vi "LED.vi"(9 "Control_State":T1, 10 "Length":dbl, 11 "Iteration_Num":dbl) -> (3 "Output_Array":u32[](array[numeric]))   [LabVIEW 2020]
uses:
  LED_Control_States.ctl
  <vilib>/numeric/Random Number (Range) U64.vi
  af1e4812-ce9e-4321-a641-5b8f74c4ca52.vi
  <vilib>/numeric/sub_Random U32.vi
panel:
  in  "Numbers":dbl[](array[numeric])=[2.0, 4.0, 100.0, 30.0, 2.0, 6.0]
  in  "colors":u32[](array[colorbox])=[16712704, 1507583, 65302]
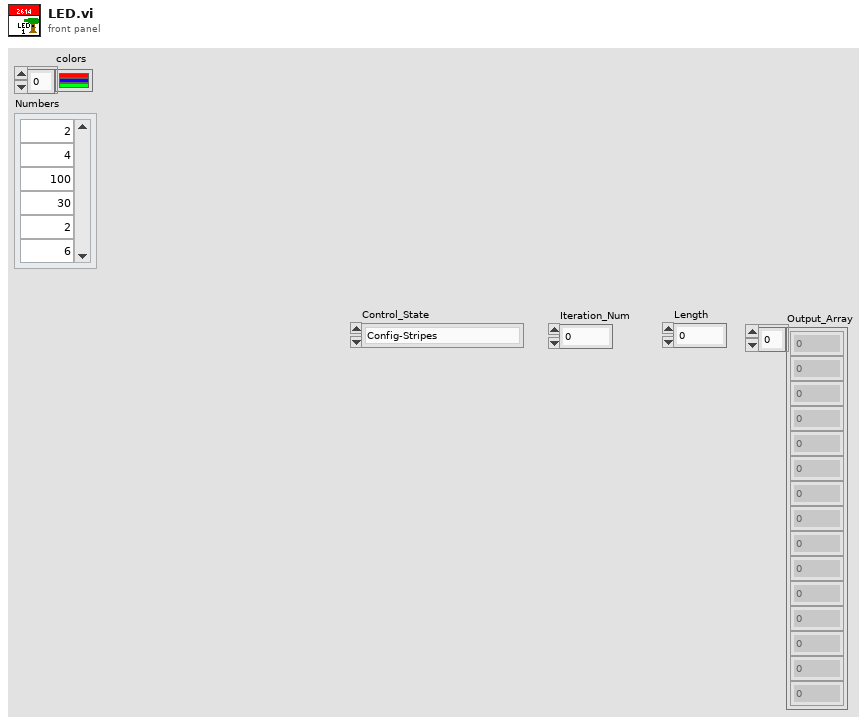
[diagram p1: front panel]
types:
  T1 = typedef "LED_Control_States.ctl" = enum16{"Config-Stripes", "swapperlines", "Rand", "Solid", "Flash-S", "Gradyent", "Move-Stripes", "Org-Rand", "Move-Point-Tail", "Flames", "Fade", "Alt-Colors"}
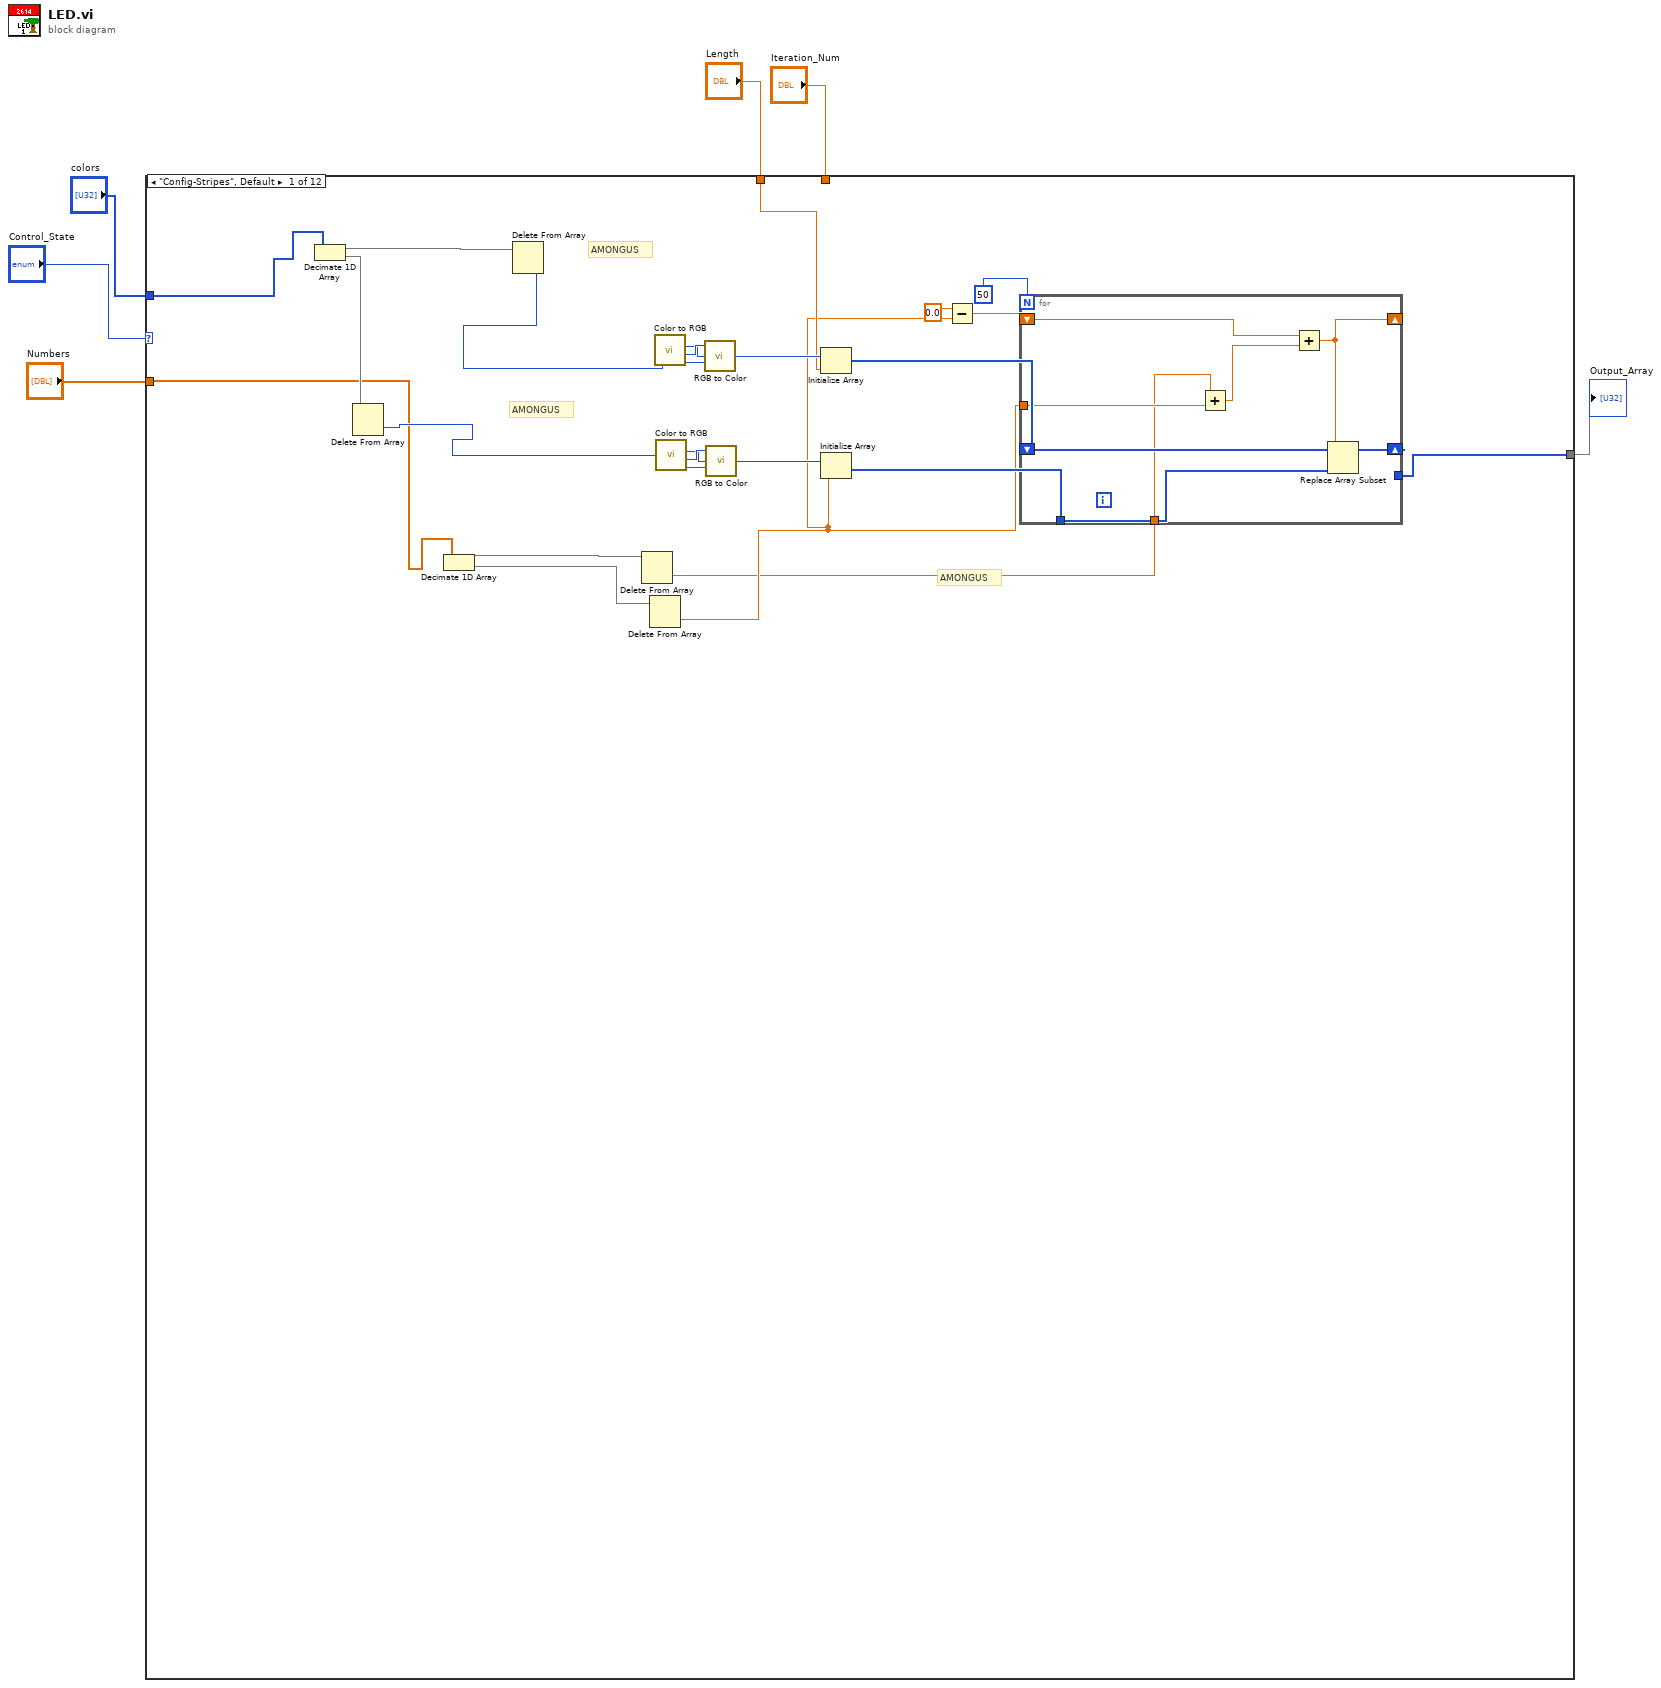
[diagram p0: block diagram]
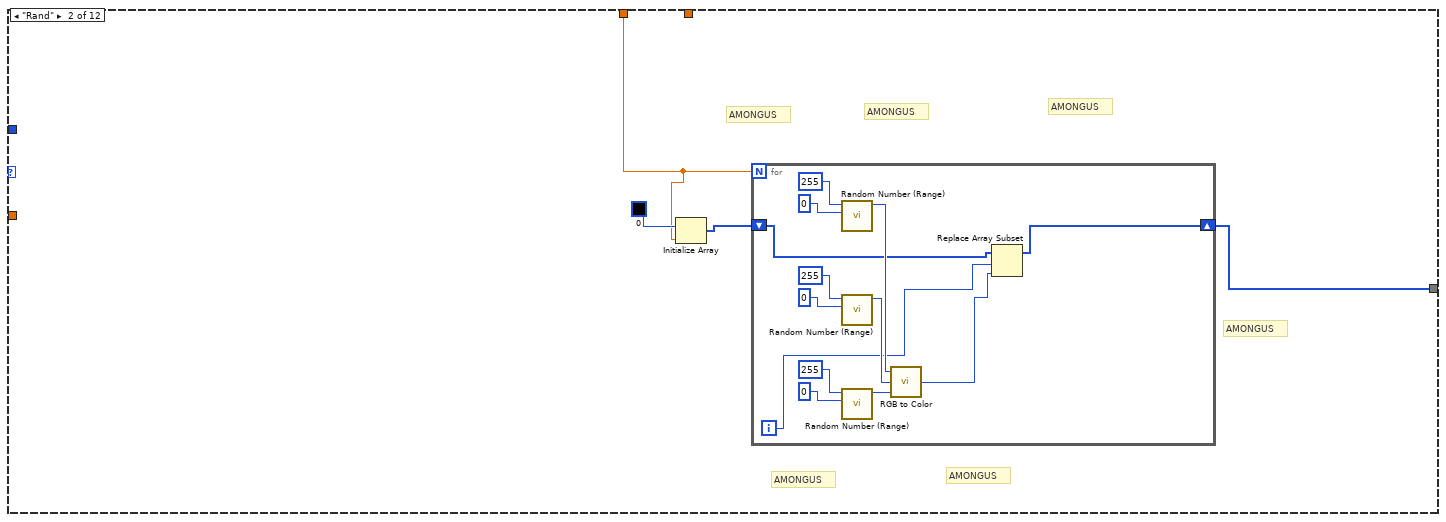
[diagram p2: hidden frame]
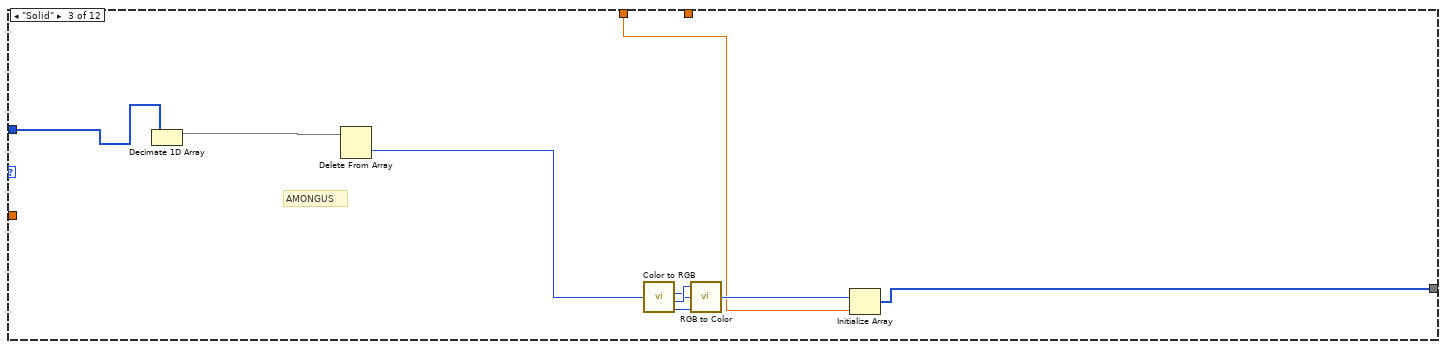
[diagram p3: hidden frame]
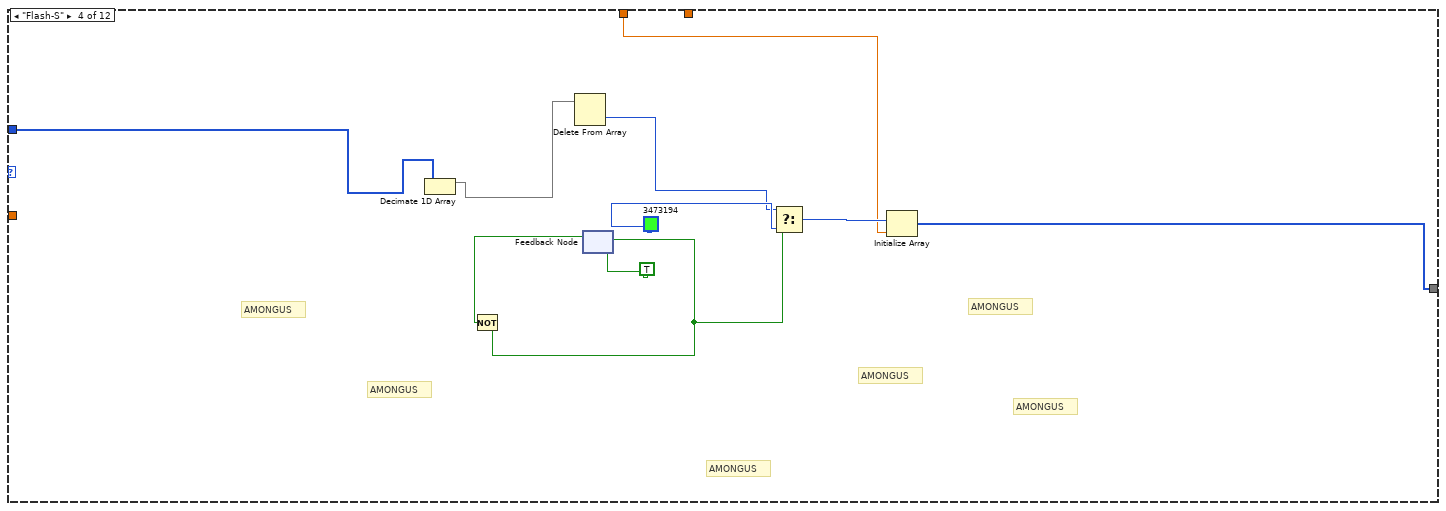
[diagram p4: hidden frame]
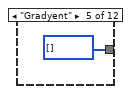
[diagram p5: hidden frame]
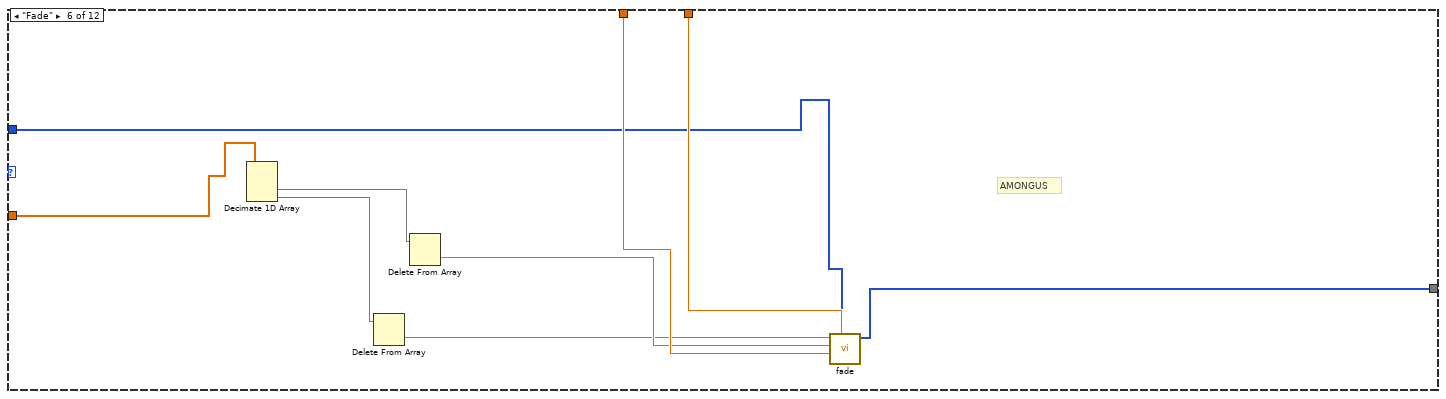
[diagram p6: hidden frame]
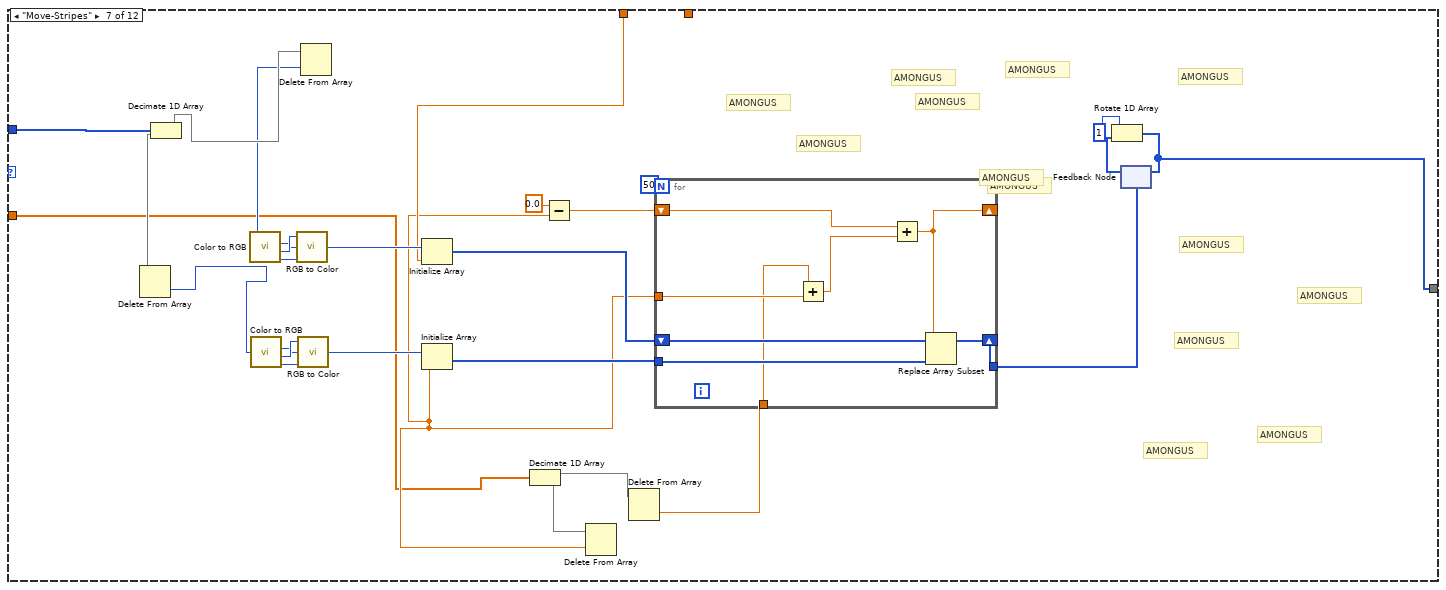
[diagram p7: hidden frame]
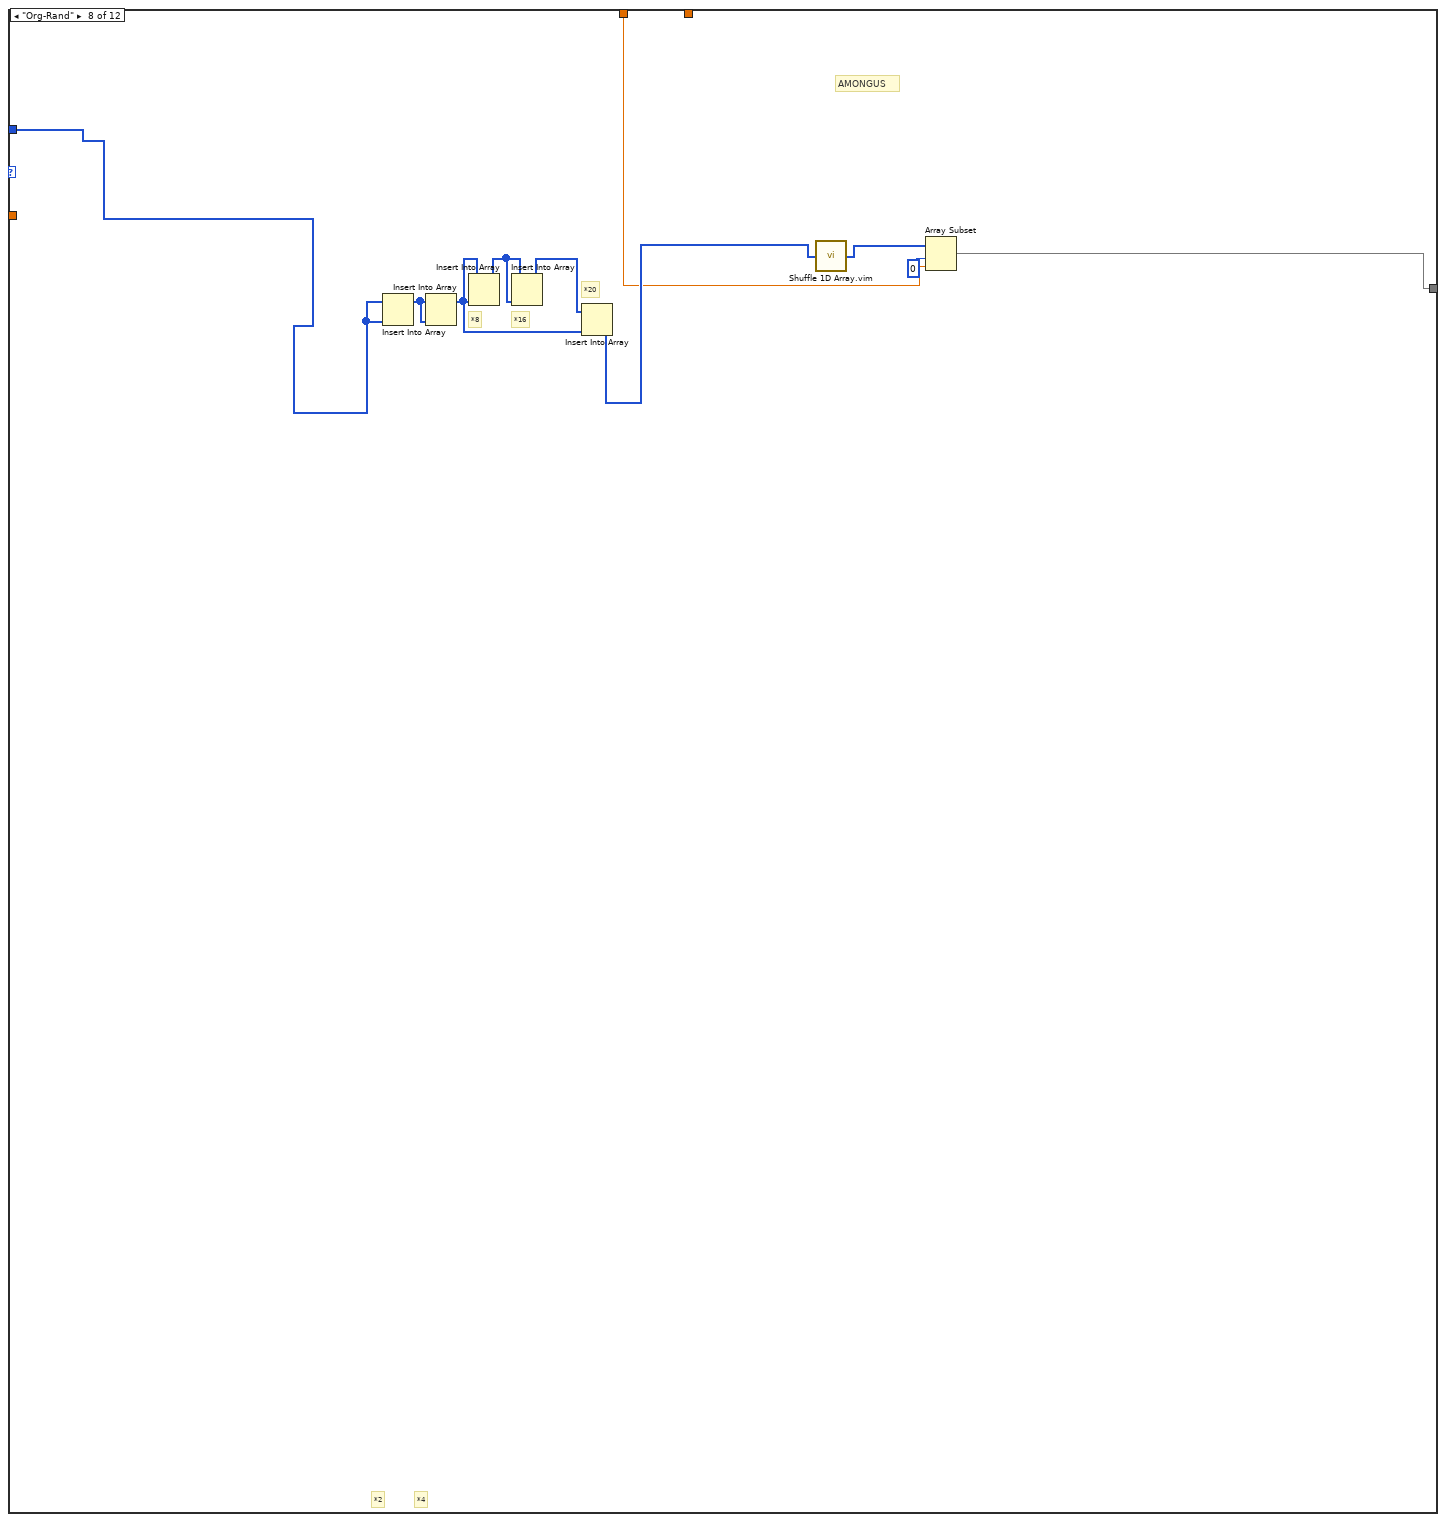
[diagram p8: hidden frame]
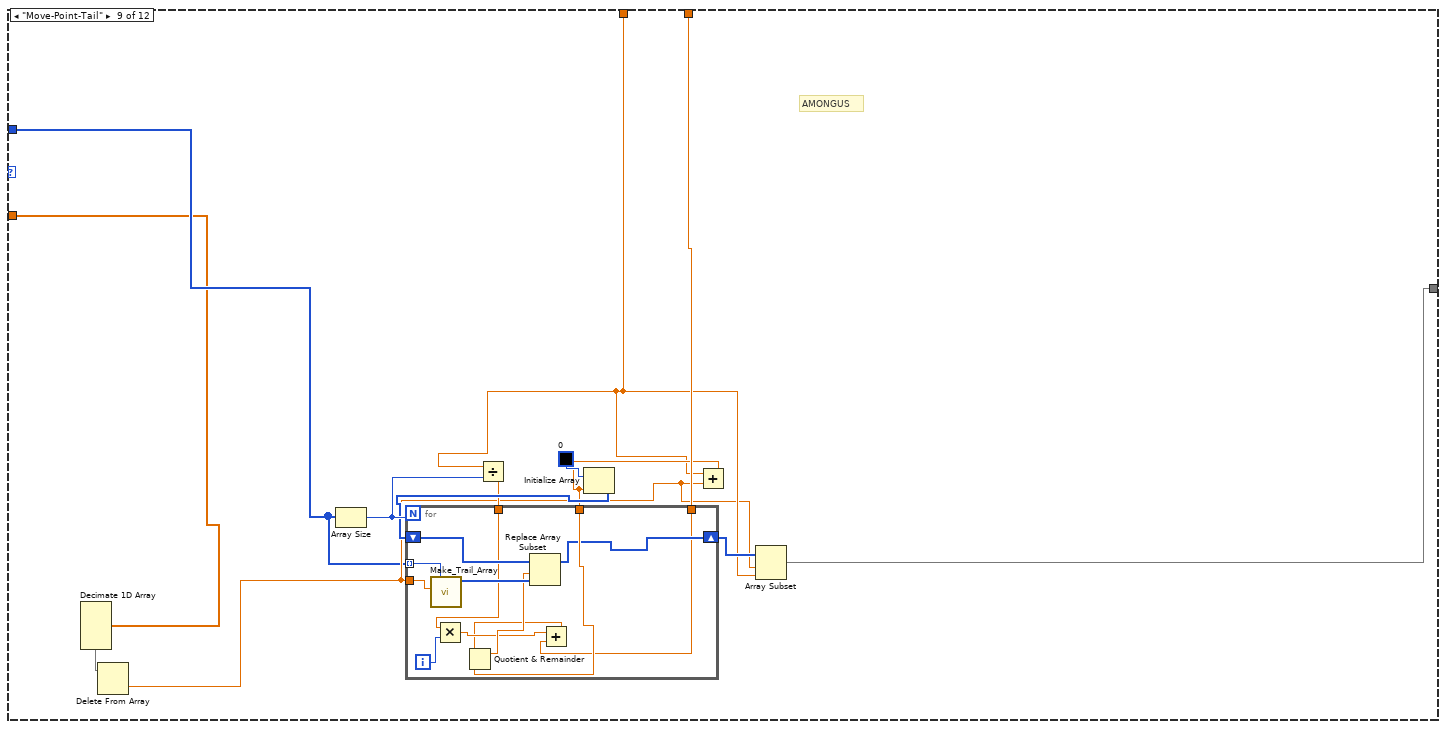
[diagram p9: hidden frame]
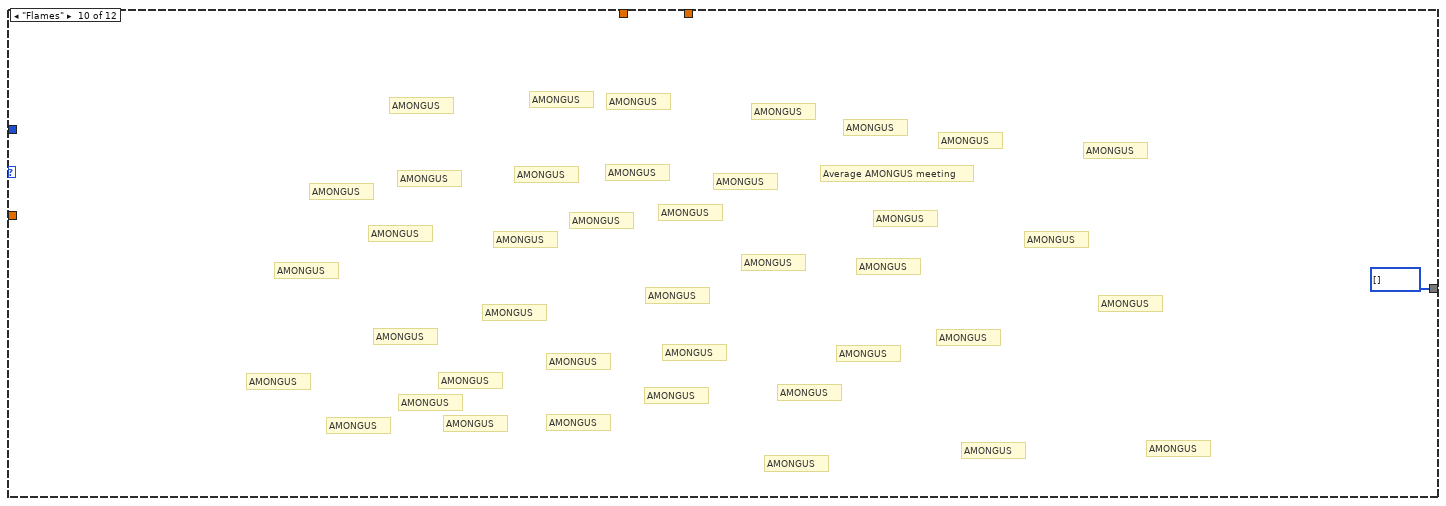
[diagram p10: hidden frame]
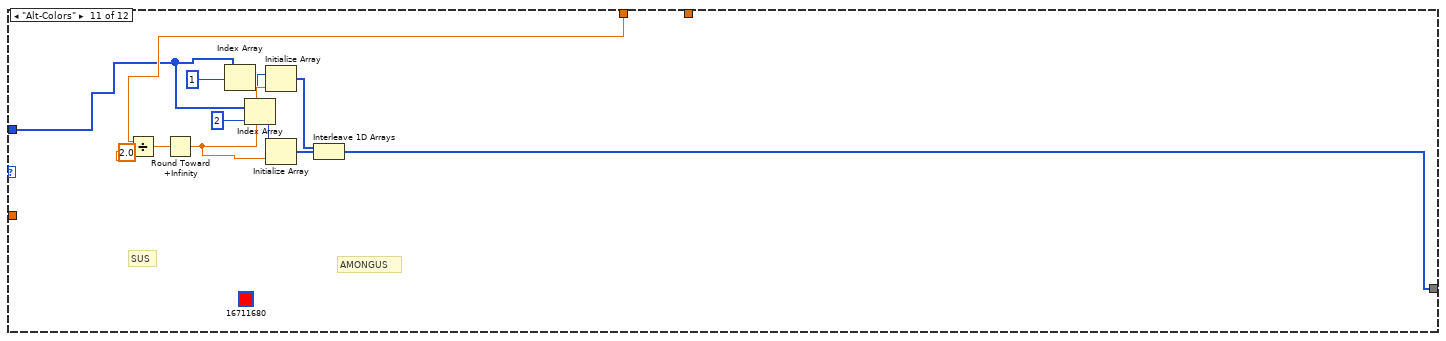
[diagram p11: hidden frame]
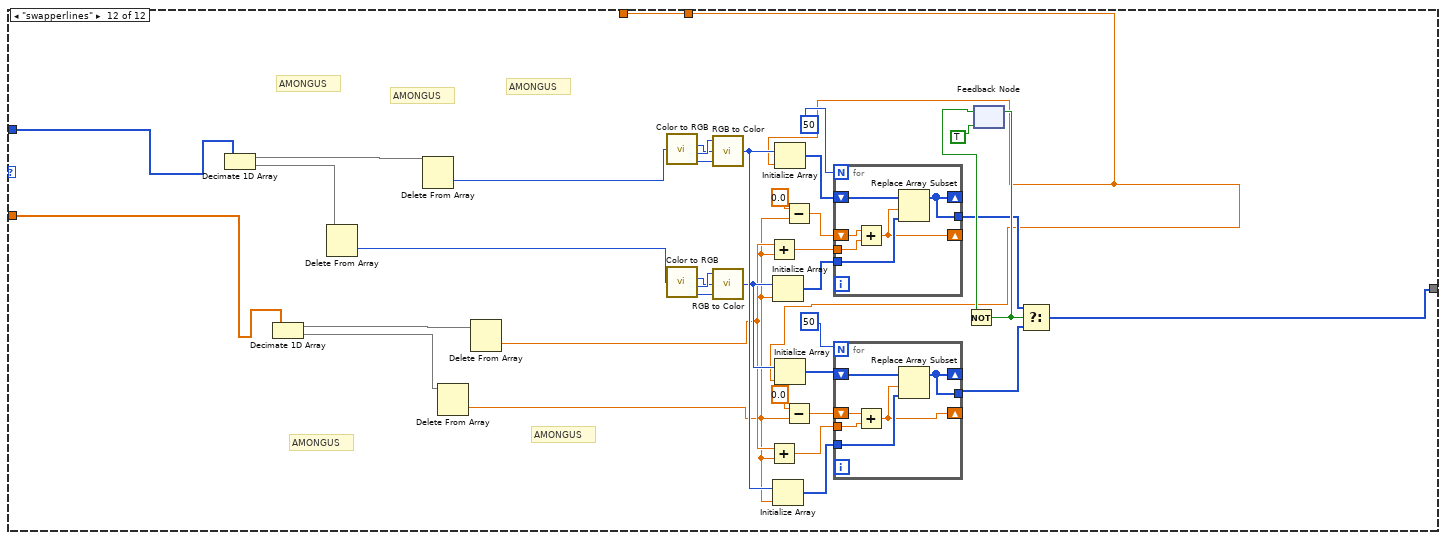
[diagram p12: hidden frame]
diagram:
  n1 = case shown="\"Config-Stripes\", Default" "Control_State" {
    tunnel: [w17 w40 w60 w69 u32[] [] ("Output_Array") w83 w96 w123 w138 u32[] [] ("Output_Array") w166 w181] -> w6
    tunnel: "Length" -> [w18 w42 w61 w70 _ w84 w100 w124 w137 _ w167 w180]
    tunnel: "Iteration_Num" -> [_ _ _ _ _ w85 _ _ w141 _ _ _]
    tunnel: "colors" -> [w8 _ w57 w66 _ w78 w87 w122 w133 _ w161 w171]
    tunnel: "Numbers" -> [w7 _ _ _ _ w77 w86 _ w132 _ _ w170]
    frame "Config-Stripes", Default {
      # "AMONGUS"
      # "AMONGUS"
      # "AMONGUS"
      n2 = Decimate 1D Array(w8) -> (w16:u32[], w15:u32[])
      n3 = Delete From Array(array=w15) -> (deleted portion=w14:u32)  [unwired: 2 in, 1 out]
      n4 = Decimate 1D Array(w7) -> (w12:dbl[], w11:dbl[])
      n5 = Delete From Array(array=w16) -> (deleted portion=w13:u32)  [unwired: 2 in, 1 out]
      n6 = Delete From Array(array=w12) -> (deleted portion=w9:dbl)  [unwired: 2 in, 1 out]
      n7 = Delete From Array(array=w11) -> (deleted portion=w10:dbl)  [unwired: 2 in, 1 out]
      n8 = call <vilib>:"Color to RGB.vi"("Color"=w13) -> ("R"=w22:u8, "G"=w23:u8, "B"=w24:u8)  [unwired: 1 out]
      n9 = call <vilib>:"Color to RGB.vi"("Color"=w14) -> ("R"=w25:u8, "G"=w26:u8, "B"=w27:u8)  [unwired: 1 out]
      n10 = call <vilib>:"RGB to Color.vi"("B"=w24, "G"=w22, "R"=w23) -> ("Color"=w21:u32)
      n11 = call <vilib>:"RGB to Color.vi"("B"=w27, "G"=w25, "R"=w26) -> ("Color"=w20:u32)
      n12 = Initialize Array(w21, w18) -> (w30:u32[])
      n13 = Initialize Array(w20, w10) -> (w19:u32[])
      n14 = Subtract(x=0.0, y=w10) -> (x-y=w28:dbl)
      n15 = for {
        N: 50 -> [_]
        shift-right: [w37] -> _
        shift-left: w28 -> [w38]
        tunnel: w19 -> [w39]
        shift-right: [w36] -> _
        shift-left: w30 -> [w35]
        tunnel: [w36] -> w17
        tunnel: w10 -> [w33]
        tunnel: w9 -> [w32]
        n16 = Add(x=w32, y=w33) -> (x+y=w34:dbl)
        n17 = Add(x=w38, y=w34) -> (x+y=w37:dbl)
        n18 = Replace Array Subset(array=w35, new element=w39, index=w37) -> (w36:u32[])
      }
    }
    frame "Rand" {
      # "AMONGUS"
      # "AMONGUS"
      # "AMONGUS"
      # "AMONGUS"
      # "AMONGUS"
      # "AMONGUS"
      n19 = Initialize Array(u32 0, w42) -> (w41:u32[])
      n20 = for {
        N: w42 -> [_]
        shift-right: [w44] -> w40
        shift-left: w41 -> [w45]
        i -> [w47]
        n21 = call-poly <vilib>:"Random Number (Range).vi"("lower bound (0)"=u64 0, "upper bound (100)"=u64 255) -> ("number"=w56:u64)  [unwired: 9 in]
        n22 = call-poly <vilib>:"Random Number (Range).vi"("lower bound (0)"=u64 0, "upper bound (100)"=u64 255) -> ("number"=w55:u64)  [unwired: 9 in]
        n23 = call-poly <vilib>:"Random Number (Range).vi"("lower bound (0)"=u64 0, "upper bound (100)"=u64 255) -> ("number"=w54:u64)  [unwired: 9 in]
        n24 = call <vilib>:"RGB to Color.vi"("B"=w54, "G"=w55, "R"=w56) -> ("Color"=w46:u32)
        n25 = Replace Array Subset(array=w45, new element=w46, index=w47) -> (w44:u32[])
      }
    }
    frame "Solid" {
      # "AMONGUS"
      n26 = Decimate 1D Array(w57) -> (w59:u32[])  [unwired: 1 out]
      n27 = Delete From Array(array=w59) -> (deleted portion=w58:u32)  [unwired: 2 in, 1 out]
      n28 = call <vilib>:"Color to RGB.vi"("Color"=w58) -> ("R"=w63:u8, "G"=w64:u8, "B"=w65:u8)  [unwired: 1 out]
      n29 = call <vilib>:"RGB to Color.vi"("B"=w65, "G"=w63, "R"=w64) -> ("Color"=w62:u32)
      n30 = Initialize Array(w62, w61) -> (w60:u32[])
    }
    frame "Flash-S" {
      # "AMONGUS"
      # "AMONGUS"
      # "AMONGUS"
      # "AMONGUS"
      # "AMONGUS"
      # "AMONGUS"
      n31 = Decimate 1D Array(w66) -> (w68:u32[])  [unwired: 1 out]
      n32 = Delete From Array(array=w68) -> (deleted portion=w67:u32)  [unwired: 2 in, 1 out]
      n33 = feedback #1(TRUE) -> (w73:bool)
      n34 = Not(x=w73) -> (.not. x?=w72:bool)
      n35 = feedback-in #1(w72) -> ()
      n36 = Select(t=w67, s=w72, f=u32 3473194) -> (s? t:f=w75:u32)
      n37 = Initialize Array(w75, w70) -> (w69:u32[])
    }
    frame "Gradyent" {
    }
    frame "Fade" {
      # "AMONGUS"
      n38 = Decimate 1D Array(w77) -> (w82:dbl[], w80:dbl[])  [unwired: 3 out]
      n39 = Delete From Array(array=w80) -> (deleted portion=w79:dbl)  [unwired: 2 in, 1 out]
      n40 = Delete From Array(array=w82) -> (deleted portion=w81:dbl)  [unwired: 2 in, 1 out]
      n41 = call "fade.vi"("Iteration_Num"=w85, "Color Array"=w78, "Length"=w84, "fade constant"=w81, "Wait_Constant"=w79) -> ("Output_Array"=w83:u32[])  [unwired: 6 in]
    }
    frame "Move-Stripes" {
      # "AMONGUS"
      # "AMONGUS"
      # "AMONGUS"
      # "AMONGUS"
      # "AMONGUS"
      # "AMONGUS"
      # "AMONGUS"
      # "AMONGUS"
      # "AMONGUS"
      # "AMONGUS"
      # "AMONGUS"
      # "AMONGUS"
      # "AMONGUS"
      n42 = Decimate 1D Array(w87) -> (w95:u32[], w92:u32[])
      n43 = Delete From Array(array=w92) -> (deleted portion=w93:u32)  [unwired: 2 in, 1 out]
      n44 = call <vilib>:"Color to RGB.vi"("Color"=w93) -> ("R"=w107:u8, "G"=w108:u8, "B"=w109:u8)  [unwired: 1 out]
      n45 = call <vilib>:"RGB to Color.vi"("B"=w109, "G"=w107, "R"=w108) -> ("Color"=w102:u32)
      n46 = Delete From Array(array=w95) -> (deleted portion=w94:u32)  [unwired: 2 in, 1 out]
      n47 = call <vilib>:"Color to RGB.vi"("Color"=w94) -> ("R"=w104:u8, "G"=w105:u8, "B"=w106:u8)  [unwired: 1 out]
      n48 = call <vilib>:"RGB to Color.vi"("B"=w106, "G"=w104, "R"=w105) -> ("Color"=w103:u32)
      n49 = Initialize Array(w103, w100) -> (w112:u32[])
      n50 = Decimate 1D Array(w86) -> (w91:dbl[], w90:dbl[])
      n51 = Delete From Array(array=w90) -> (deleted portion=w89:dbl)  [unwired: 2 in, 1 out]
      n52 = Initialize Array(w102, w89) -> (w101:u32[])
      n53 = Subtract(x=0.0, y=w89) -> (x-y=w110:dbl)
      n54 = Delete From Array(array=w91) -> (deleted portion=w88:dbl)  [unwired: 2 in, 1 out]
      n55 = for {
        N: 50 -> [_]
        shift-right: [w119] -> _
        shift-left: w110 -> [w120]
        tunnel: w101 -> [w121]
        shift-right: [w118] -> _
        shift-left: w112 -> [w117]
        tunnel: [w118] -> w99
        tunnel: w89 -> [w115]
        tunnel: w88 -> [w114]
        n56 = Add(x=w114, y=w115) -> (x+y=w116:dbl)
        n57 = Add(x=w120, y=w116) -> (x+y=w119:dbl)
        n58 = Replace Array Subset(array=w117, new element=w121, index=w119) -> (w118:u32[])
      }
      n59 = feedback #2(w99) -> (w97:u32[])
      n60 = Rotate 1D Array(1:w97, 2:1 ("n")) -> (0:w96:u32[])
      n61 = feedback-in #2(w96) -> ()
    }
    frame "Org-Rand" {
      # "AMONGUS"
      # "*20"
      # "*16"
      # "*8"
      # "*4"
      # "*2"
      n62 = Insert Into Array(array=w122, new element=w122) -> (w131:u32[])  [unwired: 1 in]
      n63 = Insert Into Array(array=w131, new element=w131) -> (w129:u32[])  [unwired: 1 in]
      n64 = Insert Into Array(array=w129, new element=w129) -> (w130:u32[])  [unwired: 1 in]
      n65 = Insert Into Array(array=w130, new element=w130) -> (w128:u32[])  [unwired: 1 in]
      n66 = Insert Into Array(array=w128, new element=w129) -> (w127:u32[])  [unwired: 1 in]
      n67 = call "Shuffle 1D Array.vim"("array"=w127) -> ("shuffled array"=w126:u32[])  [unwired: 4 in]
      n68 = Array Subset(array=w126, index=0, length=w124) -> (w123:u32[])
    }
    frame "Move-Point-Tail" {
      # "AMONGUS"
      n69 = Decimate 1D Array(w132) -> (w135:dbl[])  [unwired: 5 out]
      n70 = Delete From Array(array=w135) -> (deleted portion=w134:dbl)  [unwired: 2 in, 1 out]
      n71 = Array Size(array=w133) -> (size(s)=w144:i32)
      n72 = Divide(x=w137, y=w144) -> (x/y=w136:dbl)
      n73 = Add(x=w137, y=w134) -> (x+y=w140:dbl)
      n74 = Initialize Array(u32 0, w140) -> (w142:u32[])
      n75 = for {
        N: w144 -> [_]
        tunnel: w133 -> [w156] mode=indexing
        shift-right: [w151] -> w139
        shift-left: w142 -> [w155]
        tunnel: w141 -> [w146]
        tunnel: w140 -> [w152]
        tunnel: w134 -> [w150]
        tunnel: w136 -> [w148]
        i -> [w149]
        n76 = call "Make_Trail_Array.vi"("Trail_Length"=w150, "Dot_Color"=w156) -> ("Trail_Array"=w154:u32[])  [unwired: 9 in]
        n77 = Multiply(x=w148, y=w149) -> (x*y=w147:dbl)
        n78 = Add(x=w147, y=w146) -> (x+y=w145:dbl)
        n79 = Quotient & Remainder(x=w145, y=w152) -> (x-y*floor(x/y)=w153:dbl)  [unwired: 1 out]
        n80 = Replace Array Subset(array=w155, new element=w154, index=w153) -> (w151:u32[])
      }
      n81 = Array Subset(array=w139, index=w134, length=w137) -> (w138:u32[])
    }
    frame "Flames" {
      # "Average AMONGUS meeting"
      # "AMONGUS"
      # "AMONGUS"
      # "AMONGUS"
      # "AMONGUS"
      # "AMONGUS"
      # "AMONGUS"
      # "AMONGUS"
      # "AMONGUS"
      # "AMONGUS"
      # "AMONGUS"
      # "AMONGUS"
      # "AMONGUS"
      # "AMONGUS"
      # "AMONGUS"
      # "AMONGUS"
      # "AMONGUS"
      # "AMONGUS"
      # "AMONGUS"
      # "AMONGUS"
      # "AMONGUS"
      # "AMONGUS"
      # "AMONGUS"
      # "AMONGUS"
      # "AMONGUS"
      # "AMONGUS"
      # "AMONGUS"
      # "AMONGUS"
      # "AMONGUS"
      # "AMONGUS"
      # "AMONGUS"
      # "AMONGUS"
      # "AMONGUS"
      # "AMONGUS"
      # "AMONGUS"
      # "AMONGUS"
      # "AMONGUS"
      # "AMONGUS"
      # "AMONGUS"
      # "AMONGUS"
      # "AMONGUS"
    }
    frame "Alt-Colors" {
      (unwired) u32 16711680
      # "SUS"
      # "AMONGUS"
      n82 = Divide(x=w167, y=2.0) -> (x/y=w165:dbl)
      n83 = Round Toward +Infinity(x=w165) -> (ceil(x): smallest int >= x=w164:dbl)
      n84 = Index Array(array=w161, index=1) -> (element=w163:u32)
      n85 = Index Array(array=w161, index=2 ("dimension size")) -> (element=w159:u32)
      n86 = Initialize Array(w163, w164) -> (w169:u32[])
      n87 = Initialize Array(w159, w164) -> (w158:u32[])
      n88 = Interleave 1D Arrays(w169, w158) -> (w166:u32[])
    }
    frame "swapperlines" {
      # "AMONGUS"
      # "AMONGUS"
      # "AMONGUS"
      # "AMONGUS"
      # "AMONGUS"
      n89 = Decimate 1D Array(w171) -> (w179:u32[], w177:u32[])
      n90 = Decimate 1D Array(w170) -> (w175:dbl[], w174:dbl[])
      n91 = Delete From Array(array=w177) -> (deleted portion=w176:u32)  [unwired: 2 in, 1 out]
      n92 = Delete From Array(array=w179) -> (deleted portion=w178:u32)  [unwired: 2 in, 1 out]
      n93 = Delete From Array(array=w174) -> (deleted portion=w172:dbl)  [unwired: 2 in, 1 out]
      n94 = Delete From Array(array=w175) -> (deleted portion=w173:dbl)  [unwired: 2 in, 1 out]
      n95 = call <vilib>:"Color to RGB.vi"("Color"=w178) -> ("R"=w187:u8, "G"=w188:u8, "B"=w189:u8)  [unwired: 1 out]
      n96 = call <vilib>:"Color to RGB.vi"("Color"=w176) -> ("R"=w183:u8, "G"=w184:u8, "B"=w185:u8)  [unwired: 1 out]
      n97 = call <vilib>:"RGB to Color.vi"("B"=w189, "G"=w187, "R"=w188) -> ("Color"=w186:u32)
      n98 = call <vilib>:"RGB to Color.vi"("B"=w185, "G"=w183, "R"=w184) -> ("Color"=w182:u32)
      n99 = Add(x=w173, y=w172) -> (x+y=w201:dbl)
      n100 = Add(x=w173, y=w172) -> (x+y=w191:dbl)
      n101 = Initialize Array(w182, w172) -> (w205:u32[])
      n102 = Initialize Array(w186, w172) -> (w195:u32[])
      n103 = Initialize Array(w186, w180) -> (w204:u32[])
      n104 = Initialize Array(w182, w180) -> (w194:u32[])
      n105 = Subtract(x=0.0, y=w172) -> (x-y=w202:dbl)
      n106 = Subtract(x=0.0, y=w172) -> (x-y=w192:dbl)
      n107 = for {
        N: 50 -> [_]
        shift-right: [w216] -> _
        shift-left: w202 -> [w217]
        tunnel: w205 -> [w218]
        shift-right: [w215] -> _
        shift-left: w204 -> [w214]
        tunnel: [w215] -> w197
        tunnel: w201 -> [w213]
        n108 = Add(x=w217, y=w213) -> (x+y=w216:dbl)
        n109 = Replace Array Subset(array=w214, new element=w218, index=w216) -> (w215:u32[])
      }
      n110 = for {
        N: 50 -> [_]
        shift-right: [w210] -> _
        shift-left: w192 -> [w211]
        tunnel: w195 -> [w212]
        shift-right: [w209] -> _
        shift-left: w194 -> [w208]
        tunnel: [w209] -> w190
        tunnel: w191 -> [w207]
        n111 = Add(x=w211, y=w207) -> (x+y=w210:dbl)
        n112 = Replace Array Subset(array=w208, new element=w212, index=w210) -> (w209:u32[])
      }
      n113 = feedback #3(TRUE) -> (w199:bool)
      n114 = Not(x=w199) -> (.not. x?=w198:bool)
      n115 = feedback-in #3(w198) -> ()
      n116 = Select(t=w197, s=w198, f=w190) -> (s? t:f=w181:u32[])
    }
  }
  "Output_Array" <- w6
